vi "Write Section - Path.vi"(4 "Relative? (F)":bool, 5 "application directory":path, 6 "Create file if not found? (T)":bool=TRUE, 7 "Value":path, 8 "error in (no error)":errorcluster, 9 "key":string, 10 "section":string, 11 "Path":path) -> (0 "error out":errorcluster)   [LabVIEW 2019, in "TSC File IO.lvlib"]
doc: "This VI will write a section/cluster configuration file with type Path.\n\nThe developer can also use this VI to write a relative path. If application directory is blank and the relative input is true, the file will be written as relative to the input ini file. If the application directory is NOT blank and the paths resolve (the file is within the app directory), then it will use the <appdir> symbolic path as the starting point for the file definition. If the file is not within the application directory input and relative is TRUE, then a hardcoded path will be written.\n\nInputs:\n-Path [path] - a path to the file\n-section [string] - the section string in the configuration file\n-key [string] - the key to be read in the configuration file\n-value [Path] - the data written\n-error in\n\nOutputs:\n-error out\n_________________________________________________________________________\n<b>Code Developed By:</b>\nDaniel Coons\nTechnology Service Corporation\n1983 S Liberty Drive\nBloomington, IN 47403\nPhone: 812 558-7100\ndaniel.coons@tsc.com\nwww.tsc.com\n\n<b>Date Created:</b> 05 SEP 2014\n<b>Date Updated:</b> 28 JUL 2021"
uses:
  TSC File IO.lvlib
  <vilib>/Utility/config.llb/NI_LVConfig.lvlib
  <vilib>/Utility/config.llb/Write Key (Path).vi
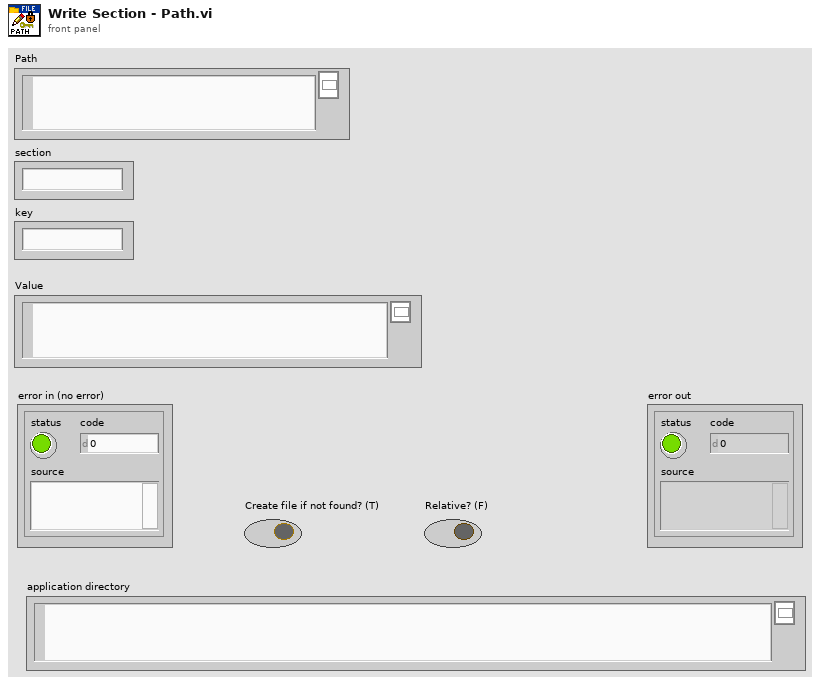
[diagram p1: front panel]
types:
  T1 = typedef "NI_LVConfig.lvlib/Config Data RefNum.ctl" = refnum<k1>
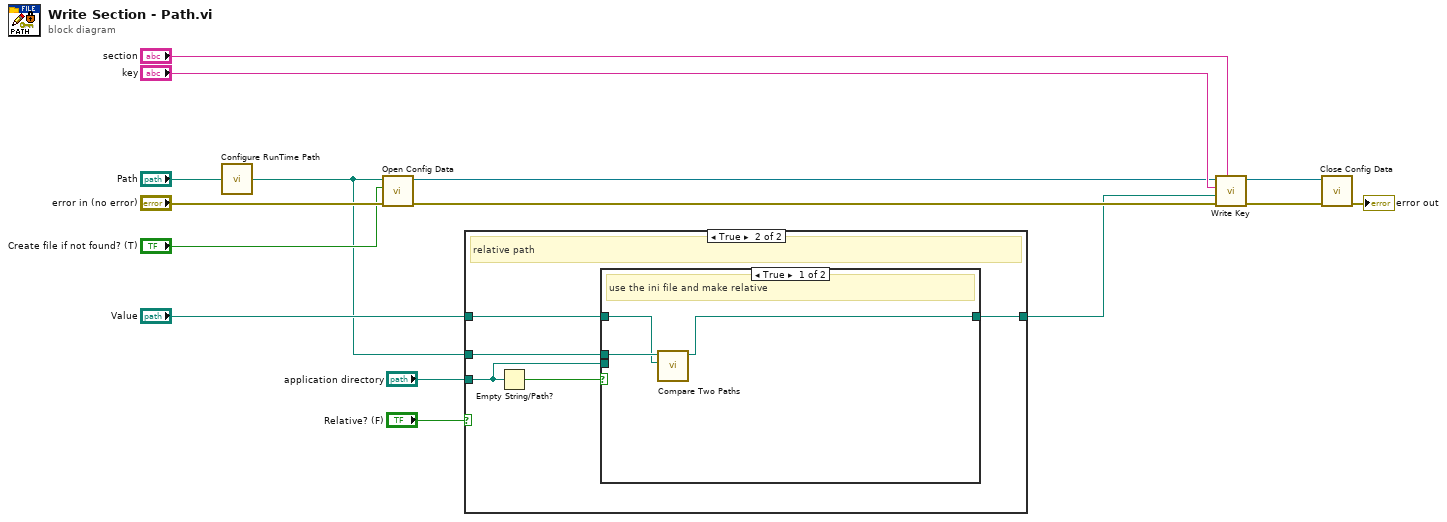
[diagram p0: block diagram]
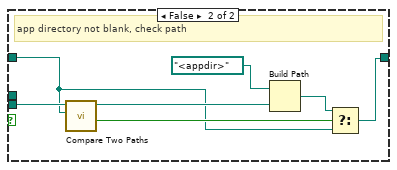
[diagram p3: hidden frame]
diagram:
  n1 = call "Configure RunTime Path.vi"("Input Path"="Path") -> ("Updated Path"=w1:path)
  n2 = call <vilib>:"Open Config Data.vi"("error in (no error)"="error in (no error)", "create file if necessary (T)"="Create file if not found? (T)", "configuration file path"=w1) -> ("error out"=w8:errorcluster, "refnum"=w9:T1)  [unwired: 6 in, 1 out]
  n3 = case shown="True" "Relative? (F)" {
    tunnel: "Value" -> [w16 w20]
    tunnel: [w16 w19] -> w3
    tunnel: "application directory" -> [_ w17]
    tunnel: w1 -> [_ w21]
    frame False {
      # "absolute path"
    }
    frame True {
      # "relative path"
      n4 = Empty String/Path?(string/path=w17) -> (empty?=w18:bool)
      n5 = case shown="True" w18 {
        tunnel: w21 -> [w24 _]
        tunnel: w20 -> [w23 w25]
        tunnel: [w22 w26] -> w19
        tunnel: w17 -> [_ w31]
        frame True {
          # "use the ini file and make relative"
          n6 = call <vilib>:"Compare Two Paths.vi"("Path 2"=w23, "Path 1"=w24) -> ("Relative Path from 1 to 2"=w22:path)  [unwired: 6 in, 3 out]
        }
        frame False {
          # "app directory not blank, check path"
          n7 = call <vilib>:"Compare Two Paths.vi"("Path 2"=w25, "Path 1"=w31) -> ("Path 2 Relative to Path 1?"=w28:bool, "Relative Path from 1 to 2"=w29:path)  [unwired: 6 in, 2 out]
          n8 = Build Path(base path=path "<appdir>", name or relative path=w29) -> (appended path=w27:path)
          n9 = Select(t=w27, s=w28, f=w25) -> (s? t:f=w26:path)
        }
      }
    }
  }
  n10 = call-poly <vilib>:"Write Key.vi"("section"="section", "error in (no error)"=w8, "value"=w3, "key"="key", "refnum"=w9) -> ("error out"=w10:errorcluster, "refnum out"=w11:T1)  [unwired: 4 in, 1 out]
  n11 = call <vilib>:"Close Config Data.vi"("error in (no error)"=w10, "refnum"=w11) -> ("error out"=→"error out":errorcluster)  [unwired: 8 in, 1 out]
